vi "Drive Motors.vi"(0 "Motor Powers":cluster{"RMotor":dbl, "LMotor":dbl}, 1 "Enum":enum16{"Start", "Run", "End"}(ring)) -> ()   [LabVIEW 2014]
uses:
  TypeDefs/PWM Module 1.ctl
  <vilib>/Rock Robotics/SystemInterfaces/Typedef/FPGA_TypedefDigitalModule.ctl
  <vilib>/Rock Robotics/SystemInterfaces/DIO/FPGA_DIOPWMChannel.ctl
  <vilib>/Rock Robotics/SystemInterfaces/DIO/FPGA_DIORelayChannel.ctl
  <vilib>/Rock Robotics/WPI/MotorControl/WPI_MotorControlOpen Talon.vi
  Team Code/Robot Global Data.vi
panel:
  out "Waveform Chart":cluster{"RMotor":dbl, "LMotor":dbl}(graph)
  in  "PWM Module (DIO A)":T1={"Module"=enum."Digital Module 1", "Roller"=enum."PWM 1", "Right Drive 3"=enum."PWM 2", "Right Drive 2"=enum."PWM 3", "Right Drive 1"=enum."PWM 4", "Shooter"=enum."PWM 5", "Unassigned"=enum."PWM 6", "Unassigned"=enum."PWM 7", "Left Drive 1"=enum."PWM 8", "Left Drive 2"=enum."PWM 9", "Left Drive 3"=enum."PWM 9", "Unassigned"=enum."Relay 1", "Unassigned"=enum."Relay 2", "Unassigned"=enum."Relay 3", "Unassigned"=enum."Relay 3", "Unassigned"=enum."Invalid", "Unassigned"=enum."Relay 1", "Unassigned"=enum."Relay 1", "Compressor "=enum."Relay 1"}
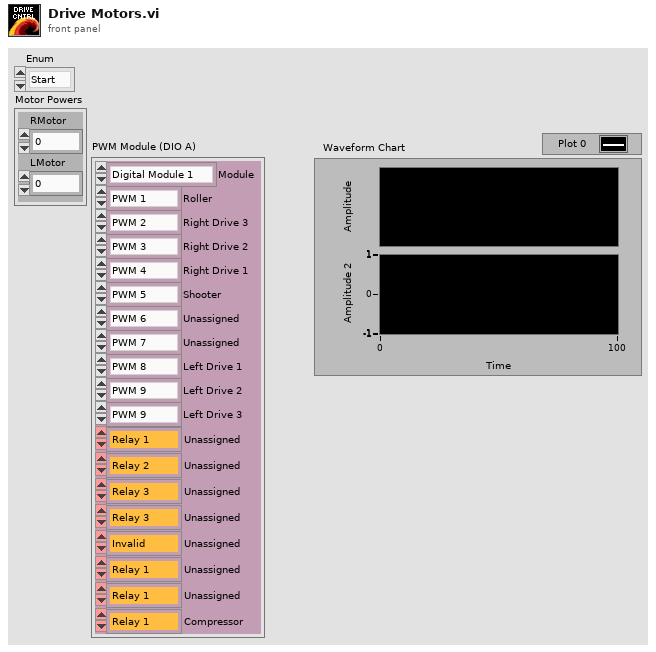
[diagram p1: front panel]
types:
  T1 = typedef "PWM Module 1.ctl" = cluster{"Module":T2, "Roller":T3, "Right Drive 3":T3, "Right Drive 2":T3, "Right Drive 1":T3, "Shooter":T3, "Unassigned":T3, "Unassigned":T3, "Left Drive 1":T3, "Left Drive 2":T3, "Left Drive 3":T3, "Unassigned":T4, "Unassigned":T4, "Unassigned":T4, "Unassigned":T4, "Unassigned":T4, "Unassigned":T4, "Unassigned":T4, "Compressor ":T4}
  T2 = typedef "FPGA_TypedefDigitalModule.ctl" = enum16{"Digital Module 1", "Digital Module 2"}
  T3 = typedef "FPGA_DIOPWMChannel.ctl" = enum8{"PWM 1", "PWM 2", "PWM 3", "PWM 4", "PWM 5", "PWM 6", "PWM 7", "PWM 8", "PWM 9", "PWM 10", "Invalid"}
  T4 = typedef "FPGA_DIORelayChannel.ctl" = enum8{"Relay 1", "Relay 2", "Relay 3", "Relay 4", "Relay 5", "Relay 6", "Relay 7", "Relay 8", "Invalid"}
  T5 = typedef "WPI_MotorControlDeviceRef.ctl" = cluster{"DeviceStatus":errorcluster, "Type":enum16{"PWM", "CAN"}, "PWM":cluster{"Digital Module":T2, "PWM Channel":T3, "DeadBand":T6}, "CAN":cluster{"Device Number":u8, "Control Mode":T7, "Semaphore":T8, "Max Vout":dbl}, "Invert":bool, "TransformRef":T9, "InvTransformRef":T9}
  T6 = typedef "WPI_PWMDeadband.ctl" = cluster{"Name":string, "maxPositivePwm":i32, "minPositivePwm":i32, "centerPwm":i32, "maxNegativePwm":i32, "minNegativePwm":i32, "angularRange":u16}
  T7 = typedef "WPI_CANJaguar_ControlMode.ctl" = enum8{"Percent VBus", "Current", "Speed", "Position", "Voltage"}
  T8 = typedef "Semaphore RefNum" = refnum<k1>
  T9 = typedef "WPI_PWMTransform_ConPane.ctl" = refnum<vi>
  T10 = cluster{"Left Power":dbl, "Right Power":dbl, "Shooter State":enum16{"Nothing", "Fire", "Load"}, "Loader State":enum16{"Loader Up", "Loader Down", "Ball In Possesion"}, "Auto Time":dbl, "Tele Time":dbl, "Driver":dbl, "Not Allowed":bool, "Right Speed":dbl, "Left Speed":dbl}
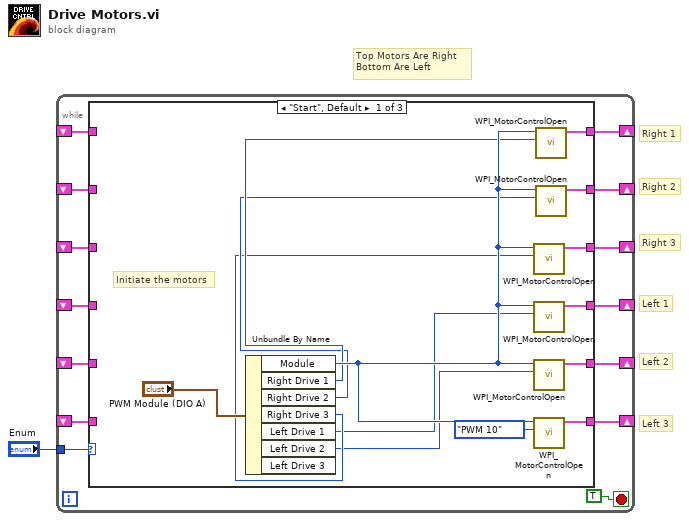
[diagram p0: block diagram]
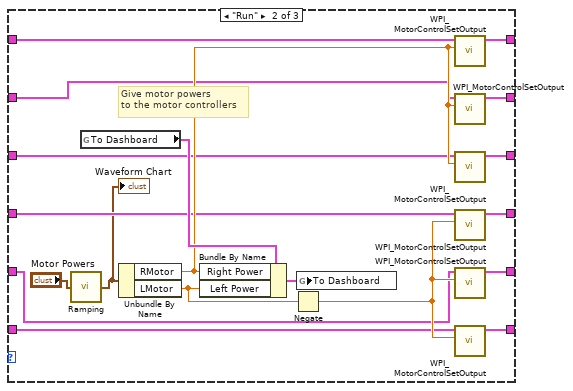
[diagram p2: hidden frame]
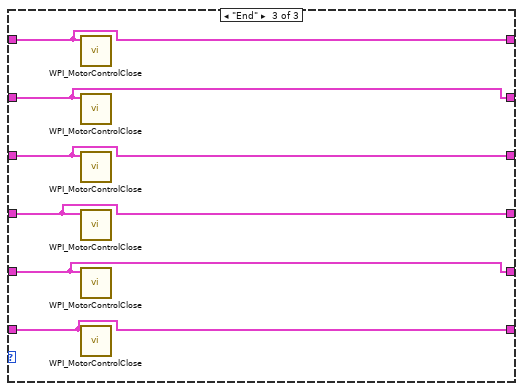
[diagram p3: hidden frame]
diagram:
  # "Left 3"
  # "Left 2"
  # "Left 1"
  # "Right 3"
  # "Right 2"
  # "Right 1"
  # "Top Motors Are Right\nBottom Are Left"
  n1 = while {
    tunnel: "Enum" -> [w14]
    shift-right: [w13] -> _
    shift-left: _ -> [w7]
    shift-right: [w12] -> _
    shift-left: _ -> [w6]
    shift-right: [w11] -> _
    shift-left: _ -> [w5]
    shift-right: [w10] -> _
    shift-left: _ -> [w4]
    shift-right: [w9] -> _
    shift-left: _ -> [w3]
    shift-right: [w8] -> _
    shift-left: _ -> [w2]
    stop <- TRUE stop-if-true
    n2 = case shown="\"Start\", Default" w14 {
      tunnel: [w22 w43 w54] -> w13
      tunnel: [w21 w45 w53] -> w12
      tunnel: [w20 w44 w52] -> w11
      tunnel: [w19 w42 w51] -> w10
      tunnel: [w18 w40 w50] -> w9
      tunnel: [w17 w41 w49] -> w8
      tunnel: w7 -> [_ w37 w54]
      tunnel: w6 -> [_ w36 w53]
      tunnel: w5 -> [_ w35 w52]
      tunnel: w4 -> [_ w34 w51]
      tunnel: w3 -> [_ w33 w50]
      tunnel: w2 -> [_ w32 w49]
      frame "Start", Default {
        # "Initiate the motors"
        n3 = Unbundle By Name("PWM Module (DIO A)") -> ("Module"=w28:T2, "Right Drive 1"=w27:T3, "Right Drive 2"=w26:T3, "Right Drive 3"=w25:T3, "Left Drive 1"=w24:T3, "Left Drive 2"=w23:T3)  [unwired: 1 out]
        n4 = call-poly <vilib>:"WPI_MotorControlOpen.vi"("PWM Channel"=w25, "Digital Module (Module 1)"=w28) -> ("MotorControlDeviceRef"=w20:T5)  [unwired: 8 in, 1 out]
        n5 = call-poly <vilib>:"WPI_MotorControlOpen.vi"("PWM Channel"=w24, "Digital Module (Module 1)"=w28) -> ("MotorControlDeviceRef"=w19:T5)  [unwired: 8 in, 1 out]
        n6 = call-poly <vilib>:"WPI_MotorControlOpen.vi"("PWM Channel"=w23, "Digital Module (Module 1)"=w28) -> ("MotorControlDeviceRef"=w18:T5)  [unwired: 8 in, 1 out]
        n7 = call-poly <vilib>:"WPI_MotorControlOpen.vi"("PWM Channel"=FPGA_DIOPWMChannel."PWM 10", "Digital Module (Module 1)"=w28) -> ("MotorControlDeviceRef"=w17:T5)  [unwired: 8 in, 1 out]
        n8 = call-poly <vilib>:"WPI_MotorControlOpen.vi"("PWM Channel"=w27, "Digital Module (Module 1)"=w28) -> ("MotorControlDeviceRef"=w22:T5)  [unwired: 8 in, 1 out]
        n9 = call-poly <vilib>:"WPI_MotorControlOpen.vi"("PWM Channel"=w26, "Digital Module (Module 1)"=w28) -> ("MotorControlDeviceRef"=w21:T5)  [unwired: 8 in, 1 out]
      }
      frame "Run" {
        # "Give motor powers\nto the motor controllers"
        n10 = call "Ramping.vi"("Motor Powers"="Motor Powers") -> ("Motor Powers"=w31:cluster{"RMotor":dbl, "LMotor":dbl})
        "Waveform Chart" <- w31
        n11 = global read "Robot Global Data.vi" "To Dashboard"() -> (w48:T10)
        n12 = Unbundle By Name(w31) -> ("RMotor"=w38:dbl, "LMotor"=w46:dbl)
        n13 = Bundle By Name(cluster=w48, "Right Power"=w38, "Left Power"=w46) -> (w47:T10)
        n14 = Negate(x=w46) -> (-x=w39:dbl)
        n15 = global write "Robot Global Data.vi" "To Dashboard"(w47) -> ()
        n16 = call <vilib>:"WPI_MotorControlSetOutput.vi"("Output"=w38, "MotorControlDevRef"=w37) -> ("MotorControlDevRef"=w43:T5)  [unwired: 7 in, 2 out]
        n17 = call <vilib>:"WPI_MotorControlSetOutput.vi"("Output"=w38, "MotorControlDevRef"=w36) -> ("MotorControlDevRef"=w45:T5)  [unwired: 7 in, 2 out]
        n18 = call <vilib>:"WPI_MotorControlSetOutput.vi"("Output"=w38, "MotorControlDevRef"=w35) -> ("MotorControlDevRef"=w44:T5)  [unwired: 7 in, 2 out]
        n19 = call <vilib>:"WPI_MotorControlSetOutput.vi"("Output"=w39, "MotorControlDevRef"=w34) -> ("MotorControlDevRef"=w42:T5)  [unwired: 7 in, 2 out]
        n20 = call <vilib>:"WPI_MotorControlSetOutput.vi"("Output"=w39, "MotorControlDevRef"=w33) -> ("MotorControlDevRef"=w40:T5)  [unwired: 7 in, 2 out]
        n21 = call <vilib>:"WPI_MotorControlSetOutput.vi"("Output"=w39, "MotorControlDevRef"=w32) -> ("MotorControlDevRef"=w41:T5)  [unwired: 7 in, 2 out]
      }
      frame "End" {
        n22 = call <vilib>:"WPI_MotorControlClose.vi"("MotorControlDevRef"=w54) -> ()  [unwired: 10 in, 1 out]
        n23 = call <vilib>:"WPI_MotorControlClose.vi"("MotorControlDevRef"=w53) -> ()  [unwired: 10 in, 1 out]
        n24 = call <vilib>:"WPI_MotorControlClose.vi"("MotorControlDevRef"=w52) -> ()  [unwired: 10 in, 1 out]
        n25 = call <vilib>:"WPI_MotorControlClose.vi"("MotorControlDevRef"=w51) -> ()  [unwired: 10 in, 1 out]
        n26 = call <vilib>:"WPI_MotorControlClose.vi"("MotorControlDevRef"=w50) -> ()  [unwired: 10 in, 1 out]
        n27 = call <vilib>:"WPI_MotorControlClose.vi"("MotorControlDevRef"=w49) -> ()  [unwired: 10 in, 1 out]
      }
    }
  }
